vi "存储Data至TDMS.vi"(8 "error in (no error)":errorcluster caption="错误输入（无错误）", 11 "TDMS":refnum<k34>) -> (0 "error out":errorcluster caption="错误输出", 3 "TDMS 2":refnum<k34>)   [LabVIEW 2018]
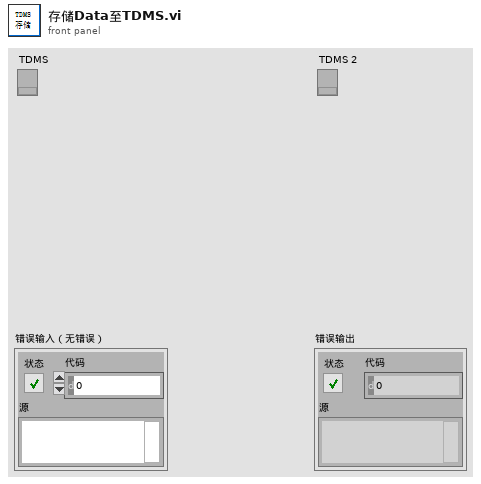
[diagram p1: front panel]
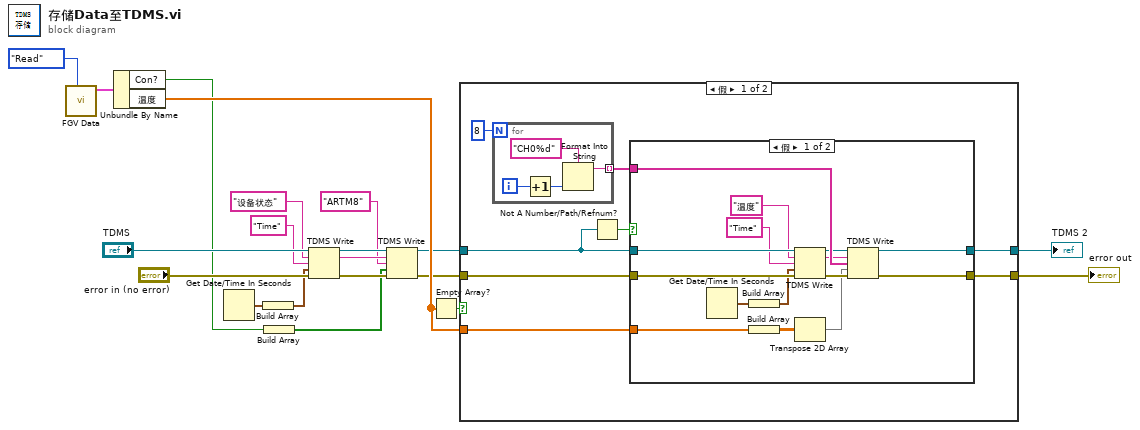
[diagram p0: block diagram]
diagram:
  n1 = call "FGV Data.vi"("Action"=enum16{"Initial", "Read", "Write"}."Read") -> ("Data OUT"=w19:cluster{"Con?":bool, "温度":dbl[]})  [unwired: 9 in, 1 out]
  n2 = Unbundle By Name(w19) -> ("Con?"=w10:bool, "温度"=w17:dbl[])
  n3 = Get Date/Time In Seconds() -> (seconds since 1Jan1904=w2:timestamp)
  n4 = Build Array(w2) -> (w1:timestamp[])
  n5 = Build Array(w10) -> (w3:bool[])
  n6 = TDMS Write(0:"TDMS", 5:"设备状态" ("组名称输入（无标题）"), 7:"Time" ("组名称输入（无标题）"), 9:w1, 11:"error in (no error)") -> (4:w9:refnum<k34>, 6:w5:string, 15:w8:errorcluster)  [unwired: 1 in, 1 out]
  n7 = TDMS Write(0:w9, 5:w5, 7:"ARTM8" ("组名称输入（无标题）"), 9:w3, 11:w8) -> (4:w7:refnum<k34>, 15:w6:errorcluster)  [unwired: 1 in, 2 out]
  n8 = Empty Array?(array=w17) -> (empty?=w15:bool)
  n9 = case shown="假" w15 {
    tunnel: [w25 w50] -> w18
    tunnel: w7 -> [w24 w51]
    tunnel: w17 -> [w23 _]
    tunnel: w6 -> [w22 w50]
    tunnel: [w21 w51] -> w16
    frame False {
      n10 = for {
        N: 8 -> [_]
        tunnel: [w29] -> w26 mode=indexing
        i -> [w32]
        n11 = Increment(x=w32) -> (x+1=w31:i32)
        n12 = Format Into String(format string="CH0%d" ("格式字符串"), w31) -> (resulting string=w29:string)  [unwired: 2 in, 1 out]
      }
      n13 = Not A Number/Path/Refnum?(number/path/refnum=w24) -> (NaN/Path/Refnum?=w28:bool)
      n14 = case shown="假" w28 {
        tunnel: w24 -> [w46 w48]
        tunnel: w23 -> [w35 _]
        tunnel: w26 -> [w47 _]
        tunnel: [w37 w49] -> w25
        tunnel: w22 -> [w39 w49]
        tunnel: [w38 w48] -> w21
        frame False {
          n15 = Get Date/Time In Seconds() -> (seconds since 1Jan1904=w44:timestamp)
          n16 = Build Array(w44) -> (w36:timestamp[])
          n17 = Build Array(w35) -> (w34:dbl[][])
          n18 = TDMS Write(0:w46, 5:"温度" ("组名称输入（无标题）"), 7:"Time" ("组名称输入（无标题）"), 9:w36, 11:w39) -> (4:w41:refnum<k34>, 6:w42:string, 15:w40:errorcluster)  [unwired: 1 in, 1 out]
          n19 = Transpose 2D Array(2D array=w34) -> (transposed array=w33:dbl[][])
          n20 = TDMS Write(0:w41, 5:w42, 7:w47, 9:w33, 11:w40) -> (4:w38:refnum<k34>, 15:w37:errorcluster)  [unwired: 1 in, 2 out]
        }
        frame True {
        }
      }
    }
    frame True {
    }
  }
  "TDMS 2" <- w16
  "error out" <- w18
